vi "Initialize.vi"(8 "error in (no error)":errorcluster, 9 "Reset (True)":bool=TRUE, 10 "ID Query (True)":bool=TRUE, 11 "VISA resource name":refnum<visa-resource-name>) -> (0 "error out":errorcluster, 1 "model":T1, 2 "idn string":string, 3 "VISA resource name out":refnum<visa-resource-name>)   [LabVIEW 2020, in "Agilent 90000 Series.lvlib"]
doc: "Establishes communication with the instrument and optionally performs an instrument identification query and/or an instrument reset. It also places the instrument in a default state needed for other instrument driver operations. Therefore, call this VI before calling other instrument driver VIs for this instrument. Generally, you need to call the Initialize VI only once at the beginning of an application."
uses:
  Agilent 90000 Series.lvlib
  Utility/DSO type.ctl
panel:
  # "(c) 2011-2014 National Instruments.  ALL RIGHTS RESERVED."
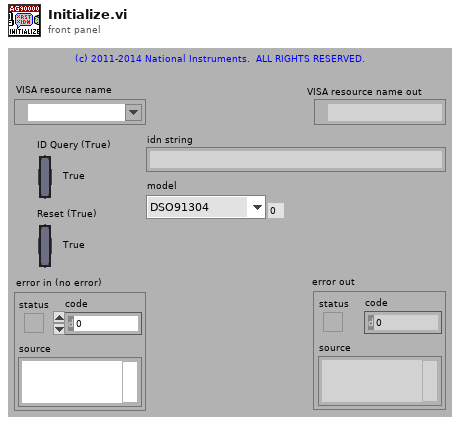
[diagram p1: front panel]
types:
  T1 = typedef "Agilent 90000 Series.lvlib/DSO type.ctl" = enum16{"DSO91304", "DSO91204", "DSO90804", "DSO90604", "DSO90404", "DSO90254", "DSA91304", "DSA91204", "DSA90804", "DSA90604", "DSA90404", "DSA90254", "DSO9104", "DSO9254", "DSO9404", "MSO9104", "MSO9254", "MSO9404", "MSO9064", "DSO9064", "DSOX91604", "DSOX92004", "DSOX92504", "DSOX92804", "DSOX93204", "DSO93004", "DSO9024H", "DSO9054H", "DSO9104H", "DSO9204H", "DSOS054A", "DSOS104A", "DSOS204A", "DSOS254A", "DSOS404A", "DSOS604A", "DSOS804A", "MSOS054A", "MSOS104A", "MSOS204A", "MSOS254A", "MSOS404A", "MSOS604A", "MSOS804A", "DSAX96204Q", "DSOX96204Q", "DSAX95004Q", "DSOX95004Q", "DSAX93304Q", "DSOX93304Q", "DSAX92504Q", "DSOX92504Q", "DSAX92004Q", "DSOX92004Q"}
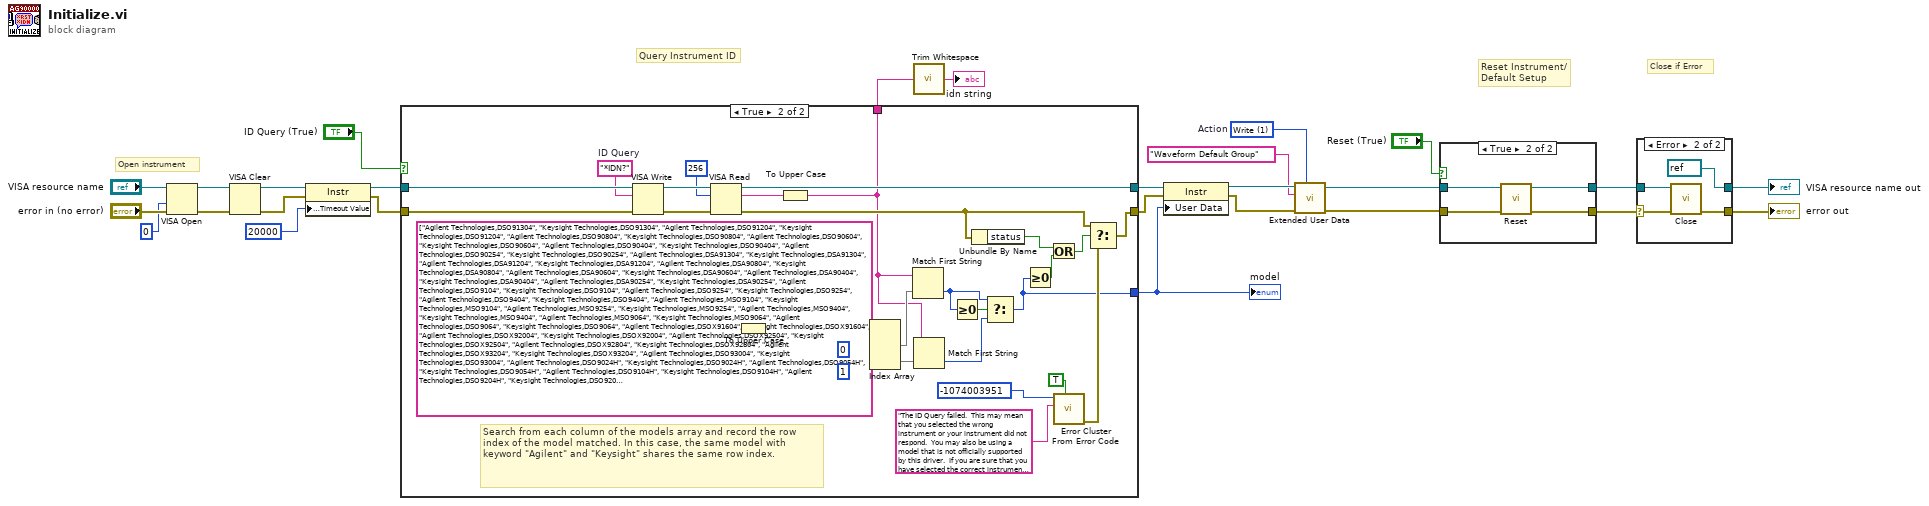
[diagram p0: block diagram]
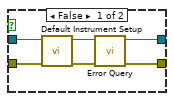
[diagram p3: hidden frame]
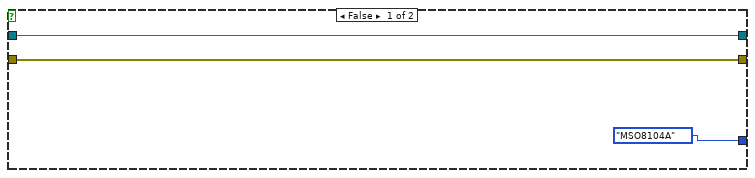
[diagram p4: hidden frame]
diagram:
  w4 = u16 1 items=["Read", "Write"]  # Action
  # "Close if Error"
  # "Query Instrument ID"
  # "Reset Instrument/\nDefault Setup"
  # "Open instrument"
  n1 = VISA Open(access mode=u32 0, error in (no error)="error in (no error)", VISA resource name="VISA resource name") -> (VISA resource name=w21:refnum<visa-resource-name>, error out=w20:errorcluster)  [unwired: 2 out]
  n2 = VISA Clear(VISA resource name=w21, error in (no error)=w20) -> (VISA resource name out=w19:refnum<visa-resource-name>, error out=w18:errorcluster)
  n3 = property on="Property Node" class="Instr"(reference=w19, error in=w18, "General Settings:Timeout Value"=u32 20000) -> (reference out=w13:refnum<visa-resource-name>, error out=w12:errorcluster)
  n4 = case shown="True" "ID Query (True)" {
    tunnel: [w29 w44] -> w11
    tunnel: [w30 w56] -> w10
    tunnel: w13 -> [w30 w57]
    tunnel: w12 -> [w29 w58]
    tunnel: [enum16{"MSO8104A"}."MSO8104A" w34] -> w1
    tunnel: [_ w32] -> w3
    frame False {
    }
    frame True {
      w52 = "*IDN?"  # ID Query
      # "Search from each column of the models array and record the row index of the model matched. In this case, the same model with keyword \"Agilent\" and \"Keysight\" shares the same row index."
      n5 = VISA Write(VISA resource name=w57, write buffer=w52, error in (no error)=w58) -> (VISA resource name out=w55:refnum<visa-resource-name>, error out=w54:errorcluster)  [unwired: 1 out]
      n6 = VISA Read(VISA resource name=w55, byte count=u32 256, error in (no error)=w54) -> (VISA resource name out=w56:refnum<visa-resource-name>, read buffer=w33:string, error out=w47:errorcluster)  [unwired: 1 out]
      n7 = To Upper Case(1:string[][] [["Agilent Technologies,DSO91304", "Keysight Technologies,DSO91304"], ["Agilent Technologies,DSO91204", "Keysight Technologies,DSO91204"], ["Agilent Technologies,DSO90804", "Keysight Technologies,DSO90804"], ["Agilent Technologies,DSO90604", "Keysight Technologies,DSO90604"], ["Agilent Technologies,DSO90404", "Keysight Technologies,DSO90404"], ["Agilent Technologies,DSO90254", "Keysight Technologies,DSO90254"], ["Agilent Technologies,DSA91304", "Keysight Technologies,DSA91304"], ["Agilent Technologies,DSA91204", "Keysight Technologies,DSA91204"], ["Agilent Technologies,DSA90804", "Keysight Technologies,DSA90804"], ["Agilent Technologies,DSA90604", "Keysight Technologies,DSA90604"], ["Agilent Technologies,DSA90404", "Keysight Technologies,DSA90404"], ["Agilent Technologies,DSA90254", "Keysight Technologies,DSA90254"], ["Agilent Technologies,DSO9104", "Keysight Technologies,DSO9104"], ["Agilent Technologies,DSO9254", "Keysight Technologies,DSO9254"], ["Agilent Technologies,DSO9404", "Keysight Technologies,DSO9404"], ["Agilent Technologies,MSO9104", "Keysight Technologies,MSO9104"], ["Agilent Technologies,MSO9254", "Keysight Technologies,MSO9254"], ["Agilent Technologies,MSO9404", "Keysight Technologies,MSO9404"], ["Agilent Technologies,MSO9064", "Keysight Technologies,MSO9064"], ["Agilent Technologies,DSO9064", "Keysight Technologies,DSO9064"], ["Agilent Technologies,DSOX91604", "Keysight Technologies,DSOX91604"], ["Agilent Technologies,DSOX92004", "Keysight Technologies,DSOX92004"], ["Agilent Technologies,DSOX92504", "Keysight Technologies,DSOX92504"], ["Agilent Technologies,DSOX92804", "Keysight Technologies,DSOX92804"], ["Agilent Technologies,DSOX93204", "Keysight Technologies,DSOX93204"], ["Agilent Technologies,DSO93004", "Keysight Technologies,DSO93004"], ["Agilent Technologies,DSO9024H", "Keysight Technologies,DSO9024H"], ["Agilent Technologies,DSO9054H", "Keysight Technologies,DSO9054H"], ["Agilent Technologies,DSO9104H", "Keysight Technologies,DSO9104H"], ["Agilent Technologies,DSO9204H", "Keysight Technologies,DSO9204H"], ["Agilent Technologies,DSOS054A", "Keysight Technologies,DSOS054A"], ["Agilent Technologies,DSOS104A", "Keysight Technologies,DSOS104A"], ["Agilent Technologies,DSOS204A", "Keysight Technologies,DSOS204A"], ["Agilent Technologies,DSOS254A", "Keysight Technologies,DSOS254A"], ["Agilent Technologies,DSOS404A", "Keysight Technologies,DSOS404A"], ["Agilent Technologies,DSOS604A", "Keysight Technologies,DSOS604A"], ["Agilent Technologies,DSOS804A", "Keysight Technologies,DSOS804A"], ["Agilent Technologies,MSOS054A", "Keysight Technologies,MSOS054A"], ["Agilent Technologies,MSOS104A", "Keysight Technologies,MSOS104A"], ["Agilent Technologies,MSOS204A", "Keysight Technologies,MSOS204A"], ["Agilent Technologies,MSOS254A", "Keysight Technologies,MSOS254A"], ["Agilent Technologies,MSOS404A", "Keysight Technologies,MSOS404A"], ["Agilent Technologies,MSOS604A", "Keysight Technologies,MSOS604A"], ["Agilent Technologies,MSOS804A", "Keysight Technologies,MSOS804A"], ["Agilent Technologies,DSAX96204Q", "Keysight Technologies,DSAX96204Q"], ["Agilent Technologies,DSOX96204Q", "Keysight Technologies,DSOX96204Q"], ["Agilent Technologies,DSAX95004Q", "Keysight Technologies,DSAX95004Q"], ["Agilent Technologies,DSOX95004Q", "Keysight Technologies,DSOX95004Q"], ["Agilent Technologies,DSAX93304Q", "Keysight Technologies,DSAX93304Q"], ["Agilent Technologies,DSOX93304Q", "Keysight Technologies,DSOX93304Q"], ["Agilent Technologies,DSAX92504Q", "Keysight Technologies,DSAX92504Q"], ["Agilent Technologies,DSOX92504Q", "Keysight Technologies,DSOX92504Q"], ["Agilent Technologies,DSAX92004Q", "Keysight Technologies,DSAX92004Q"], ["Agilent Technologies,DSOX92004Q", "Keysight Technologies,DSOX92004Q"]] ("appended array 2")) -> (0:w31:string[][])
      n8 = To Upper Case(1:w33) -> (0:w32:string)
      n9 = Index Array(array=w31, index (col) #1=0 ("disabled index (col)"), index (col) #2=1 ("disabled index (col)")) -> (element #1=w42:string[], element #2=w39:string[])  [unwired: 2 in]
      n10 = Match First String(2:w42, 3:w32) -> (0:w37:i32)  [unwired: 1 out]
      n11 = Match First String(2:w39, 3:w32) -> (0:w36:i32)  [unwired: 1 out]
      n12 = Greater Or Equal To 0?(x=w37) -> (x >= 0?=w38:bool)
      n13 = Unbundle By Name(w47) -> ("status"=w46:bool)
      n14 = Select(t=w37, s=w38, f=w36) -> (s? t:f=w34:i32)
      n15 = Greater Or Equal To 0?(x=w34) -> (x >= 0?=w35:bool)
      n16 = Or(x=w46, y=w35) -> (x .or. y?=w45:bool)
      n17 = call <vilib>:"Error Cluster From Error Code.vi"("show call chain? (False)"=TRUE, "error message (\"\")"="The ID Query failed.  This may mean that you selected the wrong instrument or your instrument did not respond.  You may also be using a model that is not officially supported by this driver.  If you are sure that you have selected the correct instrument and it is responding, try disabling the ID Query." ("Source (VI Name)"), "error code (0)"=-1074003951 ("Code")) -> ("error out"=w51:errorcluster)  [unwired: 1 in, 5 out]
      n18 = Select(t=w47, s=w45, f=w51) -> (s? t:f=w44:errorcluster)
    }
  }
  "model" <- w1
  n19 = call <vilib>:"Trim Whitespace.vi"("string"=w3) -> ("trimmed string"=→"idn string":string)  [unwired: 1 in]
  n20 = property on="Property Node" class="Instr"(reference=w10, error in=w11, "User Data"=w1) -> (reference out=w9:refnum<visa-resource-name>, error out=w8:errorcluster)
  n21 = call "Extended User Data.vi"("Action"=w4, "Error In (no error)"=w8, "Default Group Name In"="Waveform Default Group", "VISA resource name in"=w9) -> ("Error Out"=w7:errorcluster, "VISA resource name out"=w6:refnum<visa-resource-name>)  [unwired: 6 out]
  n22 = case shown="True" "Reset (True)" {
    tunnel: w7 -> [w63 w65]
    tunnel: [w60 w68] -> w14
    tunnel: w6 -> [w64 w66]
    tunnel: [w61 w67] -> w15
    frame False {
      n23 = call "Default Instrument Setup.vi"("error in (no error)"=w63, "VISA resource name"=w64) -> ("error out"=w59:errorcluster, "VISA resource name out"=w62:refnum<visa-resource-name>)  [unwired: 8 out]
      n24 = call "Error Query.vi"("error in (no error)"=w59, "VISA resource name"=w62) -> ("error out"=w60:errorcluster, "VISA resource name out"=w61:refnum<visa-resource-name>)  [unwired: 8 out]
    }
    frame True {
      n25 = call "Reset.vi"("error in (no error)"=w65, "VISA resource name"=w66) -> ("error out"=w68:errorcluster, "VISA resource name out"=w67:refnum<visa-resource-name>)  [unwired: 8 out]
    }
  }
  n26 = case shown="Error" w14 {
    selector: w14 -> [w69 w72]
    tunnel: w15 -> [w70 w73]
    tunnel: [w70 refnum<visa-resource-name> refnum ("VISA resource name out")] -> w17
    tunnel: [w69 w74] -> w16
    frame No Error {
    }
    frame Error {
      n27 = call "Close.vi"("error in (no error)"=w72, "VISA resource name"=w73) -> ("error out"=w74:errorcluster)  [unwired: 9 out]
    }
  }
  "VISA resource name out" <- w17
  "error out" <- w16
